vi "Win32-GetWindowRect.vi"(4 "error in (no error)":errorcluster, 6 "Window Name":string="EPhys Analysis", 7 "VI reference":refnum<vi>) -> (0 "error out":errorcluster, 1 "window rect":T1)   [LabVIEW 2015]
doc: "This VI will find the coordinates of the upper left and lower right corners of the window identified by the 'window refnum' parameter. Coordinate values are in pixels, relative to the upper left corner of the screen. The 'window refnum' can be obtained by using 'Get Window RefNum.vi'."
uses:
  C:/Users/hancock/Desktop/WINUTIL.LLB/Window Rectangle.ctl
  user32.dll
  kernel32.dll
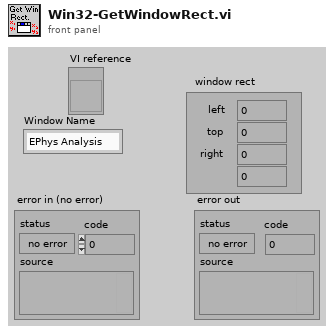
[diagram p1: front panel]
types:
  T1 = typedef "Window Rectangle.ctl" = cluster{"left":i16, "top":i16, "right":i16, "bottom":i16}
  T2 = cluster{"RECT[0]":i32, "RECT[1]":i32, "RECT[2]":i32, "RECT[3]":i32}
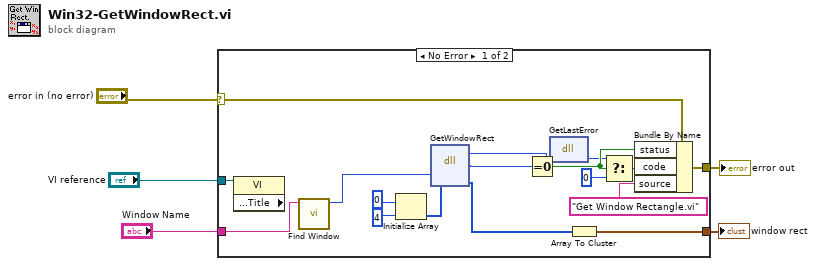
[diagram p0: block diagram]
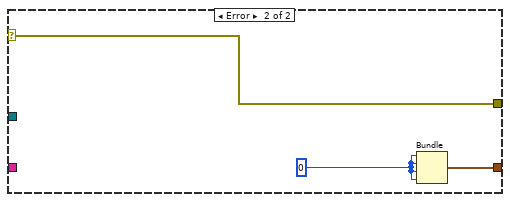
[diagram p2: hidden frame]
diagram:
  n1 = case shown="No Error" "error in (no error)" {
    selector: "error in (no error)" -> [w20 w24]
    tunnel: [w19 w24] -> w4
    tunnel: [w12 w23] -> w3
    tunnel: "VI reference" -> [w8 _]
    tunnel: "Window Name" -> [w6 _]
    frame No Error {
      n2 = property class="VI" props=["Front Panel.Title"](reference=w8) -> ()  [unwired: 1 in, 3 out]
      n3 = call "Find Window.vi"("Window Name"=w6) -> ("Win32 Window Handle"=w7:i32)  [unwired: 9 in, 1 out]
      n4 = Initialize Array(0, 4) -> (w16:i32[])
      n5 = dll-call lib="USER32.DLL" fn="GetWindowRect"("hWnd"=w7, "RECT"=w16) -> ("Return Value"=w10:i32, "RECT"=w13:i32[])  [unwired: 4 in, 2 out]
      n6 = Equal To 0?(x=w10) -> (x = 0?=w11:bool)
      n7 = dll-call lib="kernel32.dll" fn="GetLastError"(w10) -> (w9:i32)  [unwired: 2 in, 2 out]
      n8 = Array To Cluster(array=w13) -> (cluster=w12:T2)
      n9 = Select(t=w9, s=w11, f=0) -> (s? t:f=w15:i32)
      n10 = Bundle By Name(cluster=w20, "status"=w11, "code"=w15, "source"="Get Window Rectangle.vi") -> (w19:errorcluster)
    }
    frame Error {
      w22 = i16 0
      n11 = Bundle(w22, w22, w22, w22) -> (w23:cluster{i16, i16, i16, i16})  [unwired: 1 in]
    }
  }
  "error out" <- w4
  "window rect" <- w3
